vi "Run Rx - Sender Port.vi"(6 "Port":u16, 8 "error in (no error)":errorcluster, 11 "Port Ref":T1) -> (0 "error out":errorcluster)   [LabVIEW 2021, in "UDP-Custom-Device Engine.lvlib"]
uses:
  UDP-Custom-Device Engine.lvlib
  <vilib>/NI/NIVS Inline Async API/_Data Access Engine/Data Access Engine/Types/Write.DVR.ctl
  <vilib>/NI/NIVS Inline Async API/_Data Access Engine/Access Type Classes/Write/Write.lvclass
  <vilib>/NI/NIVS Inline Async API/_Data Access Engine/Access Type Classes/Write/Write.lvclass/Write.ctl
  <vilib>/NI/NIVS Inline Async API/_Data Access Engine/Data Access Engine/Methods/Write.Data.vi
  <vilib>/NI VeriStand/VeriStand Data/Type Conversion/Type Conversion.To Double (U16).vi
  <vilib>/NI/NIVS Inline Async API/_Data Access Engine/Access Type Classes/Write/Write.ProcessData.vi
  <vilib>/NI/NIVS Inline Async API/_Data Access Engine/Access Type Classes/Write/Write.Buffer.vi
  <vilib>/NI/NIVS Inline Async API/_Data Access Engine/Access Type Classes/Write/Write.Commit.vi
  <vilib>/NI VeriStand/VeriStand Data/VeriStand Data.lvlib
  <vilib>/NI/NIVS Inline Async API/_Data Access Engine/Data Access Engine/Data Access Engine.lvclass
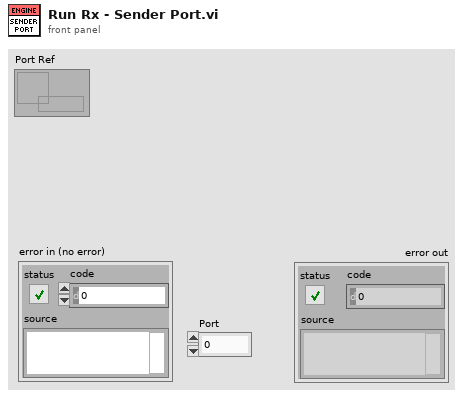
[diagram p1: front panel]
types:
  T1 = typedef "Data Access Engine.lvlib/Data Access Engine.lvclass/Write.DVR.ctl" = refnum<data-value>
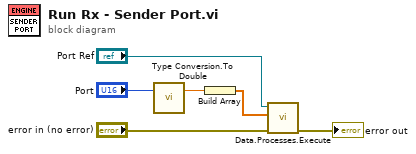
[diagram p0: block diagram]
diagram:
  n1 = call-poly <vilib>:"Type Conversion.To Double.vi"("value in"="Port") -> ("value out"=w1:dbl)  [unwired: 2 in]
  n2 = Build Array(w1) -> (w6:dbl[])
  n3 = call-poly <vilib>:"Data.Processes.Execute.vi"("error in (no error)"="error in (no error)", "Values"=w6, "Ref"="Port Ref") -> ("error out"=→"error out":errorcluster)  [unwired: 8 in]
